vi "Close.vi"(8 "error in (no error)":errorcluster, 11 "Fluke Hydra 2625A in":refnum<class "Fluke Hydra 2625A.lvclass">) -> (0 "error out":errorcluster, 3 "Fluke Hydra 2625A out":refnum<class "Fluke Hydra 2625A.lvclass">)   [LabVIEW 2014, in "Generic Data Acquisition.lvlib" / "Fluke Hydra.lvlib" / "Fluke Hydra 2625A.lvclass"]
uses:
  Fluke Hydra 2625A.lvclass
  <instrlib>/Fluke 2625A/Fluke 2625A.lvlib
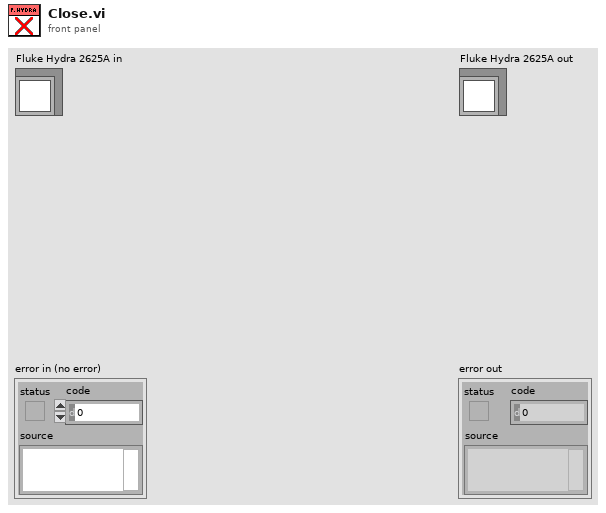
[diagram p1: front panel]
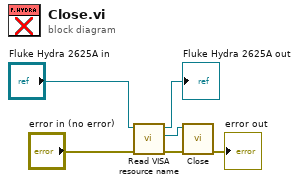
[diagram p0: block diagram]
diagram:
  n1 = call-dynamic "Read VISA resource name.vi"("error in (no error)"="error in (no error)", "Generic Instrument in"="Fluke Hydra 2625A in") -> ("error out"=w2:errorcluster, "VISA resource name"=w4:refnum<visa-resource-name>, "Generic Instrument out"=→"Fluke Hydra 2625A out":refnum<class "Fluke Hydra 2625A.lvclass">)  [unwired: 7 in]
  n2 = call <instrlib>:"Close.vi"("Error In"=w2, "VISA Resource Name In"=w4) -> ("Error Out"=→"error out":errorcluster)  [unwired: 9 in]
